vi "Main_06A.vi"() -> (3 "Set":set{cluster{i32, "index of element":i32}}(c389))   [LabVIEW 2024]
panel:
  out "2D Array":string[][](array[string])
  in  "Select Puzzle":bool
  out "Answer":u32
  in  "Puzzle":string="..........#...........#...........#.............................#......................#.........#................................\n..........................#.........#......#.................................#...........................#........................\n..................................#...#................................................................................#..........\n.#...............#.....#..........#.........#......#........#................................#......#.............................\n...#.......#.............#.............................................#.........##...............#.................#.............\n.......................................#.............#..................#........#.......#.........#...............#.........#....\n.....#..................#..#..#.........................#...................#....#........#.............................#.........\n.......#.............................#..........#......#..........................##......#.......................##..............\n.....#.....#........................................................................................#.......#.....................\n.................................#............#...#.....................................................#.........#...............\n...............#.....#..#....#....#.....................................................#............#........#.#.................\n.......#.....#...........................................................#............................#.................#....#....\n...........................#.................#....................................#...............#..#........................#...\n.....#.........................................#.................#...##....................................#......................\n.............#...#..................#......#.................#..........................................#.....#..........#........\n.................#...............#............#.......#.#...............................................#..................#......\n.....#..#.....................#.......................................................#..............#..............#.......##....\n..##........#....................................................#.............#..............#........................#..#.......\n..............................#...........#...#........................#............#..........................#........#........#\n.....................................##...............................#............#............#....#............................\n...##........................#.....#....#.........#.................................................#.............................\n...............................#................................#...............#.....#.....................#.....................\n................................................#..........#....#............................#.....#.......#..................#...\n.............#.....#.........#.#....#................##......#.............#......................................................\n..........#..............#..........#......#.........#...#.........................................#.#.....#.........#............\n..................#......................#.............................#...................#.....................................#\n................#.....#..............................#.............#.............#..#.....#....................................#..\n.........#.#................#.........#.................#...................#................................#................#...\n.............................................................#..............#.....................................................\n......#.........................#...........#.........#..................#....................................#..#...........##...\n.............................................................................#.............#........................#...#.........\n......#......#..#............#..............................................#....#..#..#................#.........#....#..........\n........#........#.........#....................................................^..#...#....................#...............#.....\n..#....#...#.......................................................................................................#..............\n.....#...........................................#..............#.........#....#........................................#.........\n.....................................#..............#............................................................#................\n.....#.......................#........................#..........#.............#.................#..................#.............\n.......................................#......#.....................................#.........................#...................\n...........................................................................................#............................##........\n..#............#..........................#...........#...#..................#......#.................#.#.................#......#\n.###......#....................#...#...........................................................#.........#.....#..............#.#.\n....................................#..........#.....#.......................#...............#.....#......#...................#...\n...#......#..................#......#.......#..............#..............#.......................................................\n..........#....................................................................#................##.#...#..........................\n.........................................................#..................##.....................#..##..........................\n..................#......#.................................#.................#.##................................................#\n...#..........#...#..#..............................................#...........................##........#.......................\n.....#................................................#...........#..................#...#.................................#......\n.......#.....#.........................#..........................................................................................\n....................................................#........#....#....................................##..............#.....#....\n............#........#.........................#.................................#..........................................#...#.\n.....................................#........................#...................#......#.#...........#..#..........#...........#\n................#...............#.........................#.........................#........#..#.................................\n.............#.........#.............#.#.#.........#...................#.......#.......................#..........................\n.............#......................................................#................................................#.......#....\n....#....................................................................#.#........#.................#..........................#\n.................................#......#....................................................................#.....#..............\n............##...................#.......................................................................#.........#........#.....\n#..................................................#..#...............#............#.............#...............................#\n.............................#.................................#.....#..........................#.............#..#...#...#........\n...#.....#..............................#.#......................................#................................................\n...#............##...............................#............#..............................#................................#...\n#.................#......##..............................................................#...........#........#...#...............\n....##.....................................................................................................#.#....................\n#.................#..................................................#..................................................#.........\n.........#.........#...........................#.................#.#.............................#................................\n................................#............#................................................................#...................\n.....................................#............................................#.##......##........#...........................\n....#....................................................#...#.#.#....................................................#...........\n.........................#.#...................#...................##...............#........................#....................\n..................................#...................................................................#.......#..................#\n...................#.............................................#.......................#.#.....................#....#...........\n#....................................#.#..#.#..........#.........#.........##.........#......................#............#.......\n...............................................................#.............................##....#.......#......................\n.............#......#.#.........#............................#............................#.......................................\n......................#.........#.........................................................#...#............#......................\n...................#.....#.....................................................#.....................................#............\n...............................#.....#..................#.......##................................................................\n.............................................#.........................#...........#..............................#..#............\n#..##..................................................................................................#......#...........#.....#.\n.......................................................#.....................#.............................#......................\n...........................................................................................................#......................\n......................#..............................................................#............................................\n...........................#.....#......................................#.........#........#..#.#.................................\n.#.......#........................................................................................................................\n.#.......#...........................................#................................#...........................................\n.........................................................#........................................#......#........................\n...............................#...#........#............................................#.................#......................\n......#.........................#......................#.....#.#..............#..................#.......#..................#.....\n.................#........#...#........................#.............................#............................................\n#...........................................................................#............................#................#.......\n..........................................................................#................#......................................\n.............#.............................................................................#.........................#............\n.#...........#.......#.......#.....#....#.......#........#....................#........................#........................#.\n...#..............#.............................#.............................................................#...#..#..........#.\n......#......#.#...............##................................................................................................#\n....#........#.##......#...#......................................................................................................\n..#..#.#.#.....................#................................#...................................#.....#...#...................\n.....................#.#........#..............##..............#.................#..............................................#.\n...................................................................................#........#.......#....#............#...........\n.....#....#..................#...............#.............................................#.#....................#...............\n.....................#..........#............#..................................#......................#.#.....#................#.\n..........#.........................................#...............#.............................................................\n.......#......................#.............#.....#..............#........................#.....#.........#.................#...#.\n..................................................................#.....#...............................................#........#\n.......#..........#.......#....#.......#..........#....#............................................#.#...........................\n..#...........#..............................#....................#....................#...#......................................\n.......#...............................#............#.....#.....................#.................................................\n.........#..................#..................#..................................................................................\n..........................................................................................#....#...................#.......##.....\n..................#.............................##.......................................................#.......#......#......#..\n...#.......#..............................................................................................#.......................\n............#..#..............................................................#...........##....#....#.#................#........#\n............#.........................#........#....#..#..................................#..................#....................\n......##......................#...##..............................#...............................................................\n........................#................#..............#...##...............................#..................##....#...........\n....#.#...#.....#..................................#..............................#...........#.....................#.............\n......................#.........................................................................#..........#.............#........\n.#......#............................................................#...............................#...#........................\n.......##.....................#.....#...........#......##.......##...................#...............................#............\n...#...#........#...............#......#......#.....#...#.................................................................#.......\n..................#.......................#...............................................#.................#.............#..#....\n.....................#.......#....#...#............................#.....................#............#.....................#.....\n................................................................#....#......#............#..................#.........#...........\n.......................#...................#..............................................................................###.....\n...............................#...........#................................#........#..#....#............................#.......\n....#......#...............................#...............#......................................#...............................\n...........#...........................##.........................................................................#.#.............\n.........................#.........#.........................................#.....#...................#.....#.......#............\n.............................#.....#................##..#.....................#..................................................."
  in  "Example":string="....#.....\n.........#\n..........\n..#.......\n.......#..\n..........\n.#..^.....\n........#.\n#.........\n......#..."
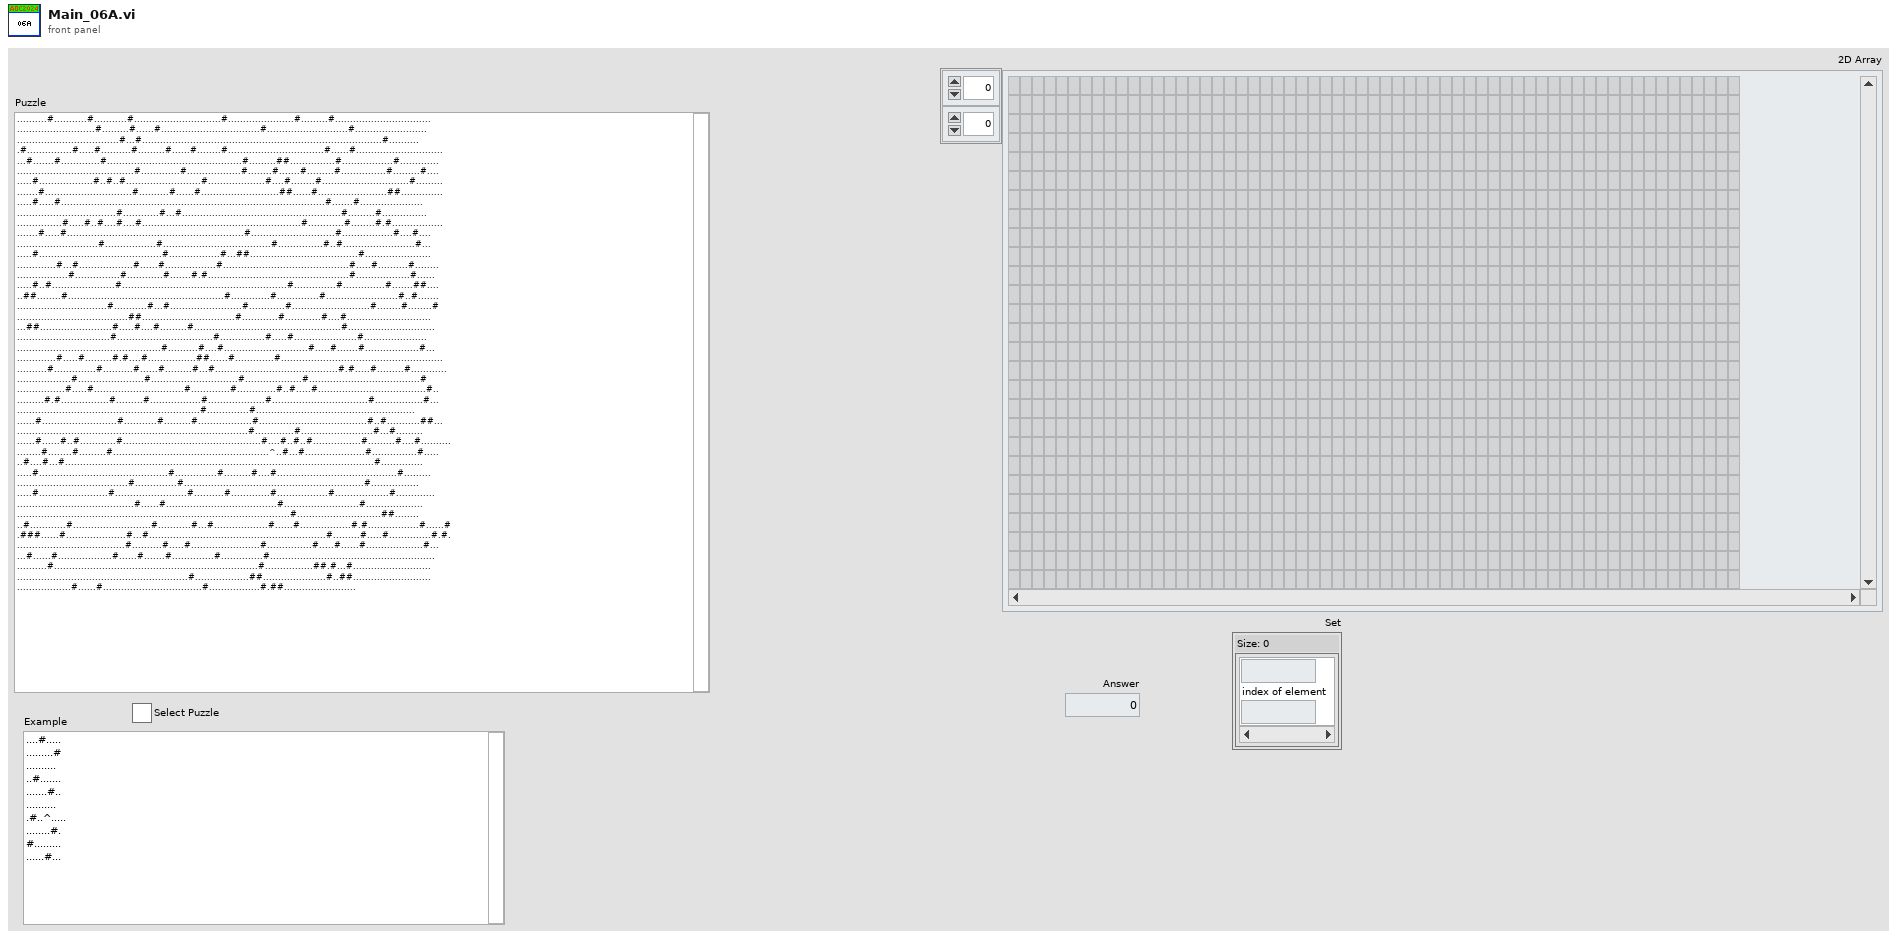
[diagram p1: front panel]
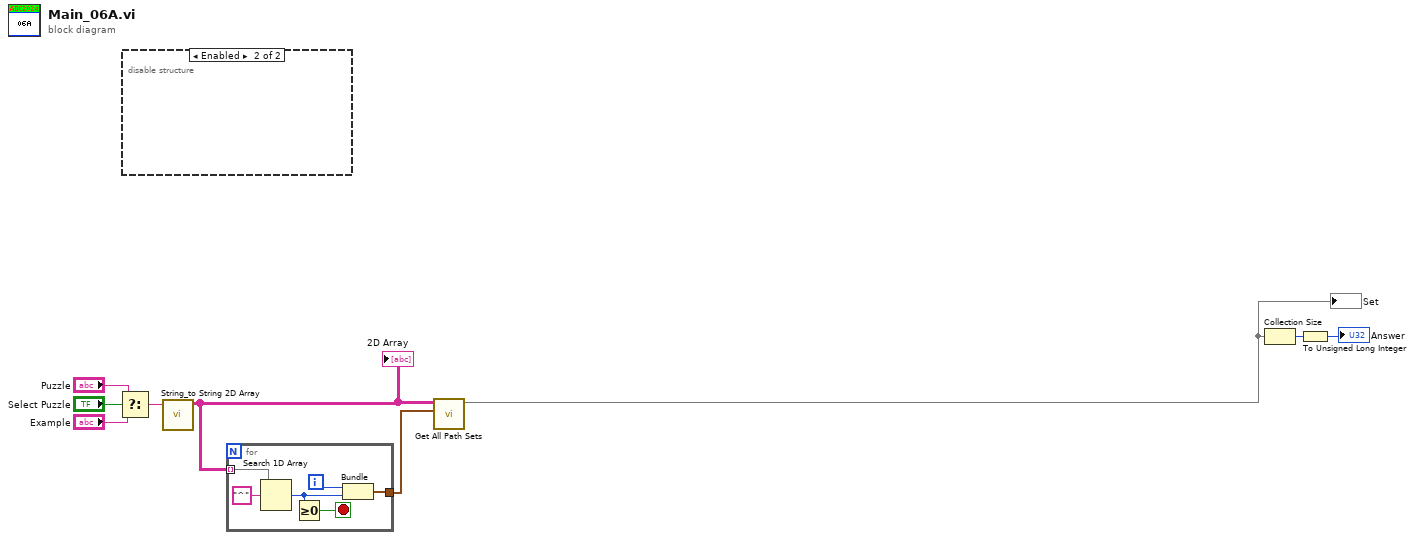
[diagram p0: block diagram]
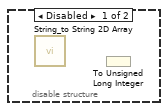
[diagram p2: hidden frame]
diagram:
  n1 = Select(t="Puzzle", s="Select Puzzle", f="Example") -> (s? t:f=w6:string)
  n2 = disable-structure shown="Enabled" {
    frame Disabled {
      n3 = call "String_to String 2D Array.vi"() -> ()  [unwired: 11 in, 1 out]
      n4 = To Unsigned Long Integer() -> ()  [unwired: 1 in, 1 out]
    }
    frame Enabled {
    }
  }
  n5 = call "String_to String 2D Array.vi"("Input String"=w6) -> ("2D Array"=w4:string[][])  [unwired: 10 in]
  "2D Array" <- w4
  n6 = for {
    tunnel: w4 -> [w15] mode=indexing
    tunnel: [w10] -> w5
    i -> [w12]
    stop <- w13 stop-if-true
    n7 = Search 1D Array(1D array=w15, element="^") -> (index of element=w11:i32)  [unwired: 1 in]
    n8 = Greater Or Equal To 0?(x=w11) -> (x >= 0?=w13:bool)
    n9 = Bundle(w12, "index of element"=w11) -> (w10:cluster{i32, "index of element":i32})  [unwired: 1 in]
  }
  n10 = call "Get All Path Sets.vi"("Start"=w5, "2D Array"=w4) -> ("Set"=w1:set{cluster{i32, "index of element":i32}})  [unwired: 9 in]
  "Set" <- w1
  n11 = Collection Size(1:w1) -> (0:w3:i32)
  n12 = To Unsigned Long Integer(number=w3) -> (unsigned 32bit integer=→"Answer":u32)
